vi "Main.vi"() -> ()   [LabVIEW 2017]
panel:
  out "Loop Run Time (ms) 2":u32
  in  "stop":bool
  out "Loop Run Time (ms)":u32
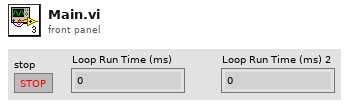
[diagram p1: front panel]
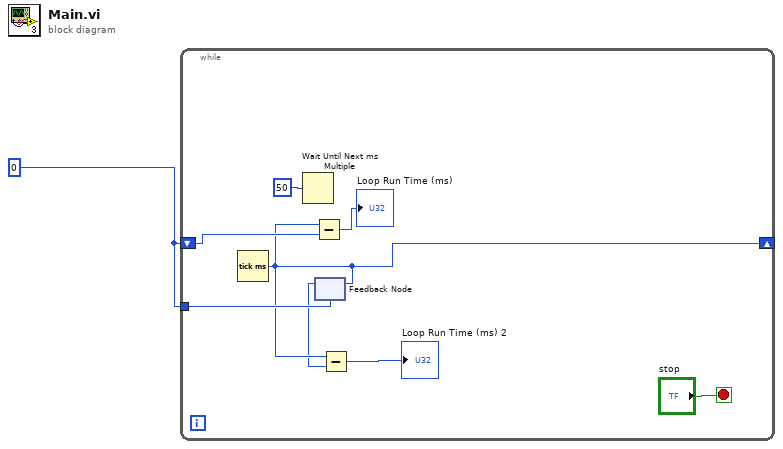
[diagram p0: block diagram]
diagram:
  w1 = u32 0
  n1 = while {
    shift-right: [w3] -> _
    shift-left: w1 -> [w6]
    tunnel: w1 -> [w5]
    stop <- "stop" stop-if-true
    n2 = Tick Count (ms)() -> (millisecond timer value=w3:u32)
    n3 = Wait Until Next ms Multiple(millisecond multiple=u32 50) -> ()  [unwired: 1 out]
    n4 = Subtract(x=w3, y=w6) -> (x-y=→"Loop Run Time (ms)":u32)
    n5 = feedback-in #1(w3) -> ()
    n6 = feedback #1(w5) -> (w2:u32)
    n7 = Subtract(x=w3, y=w2) -> (x-y=→"Loop Run Time (ms) 2":u32)
  }
